vi "From Notification Key.vi"(2 "Key":string) -> (5 "Alias":string, 8 "Symbol Name":string)   [LabVIEW 2018, in "TwinCAT ADS.lvclass"]
uses:
  TwinCAT ADS.lvclass
  Controls/ADS Notification Map Key.ctl
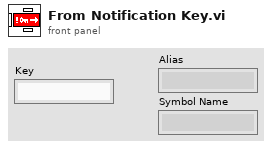
[diagram p1: front panel]
types:
  T1 = typedef "TwinCAT ADS.lvclass/ADS Notification Map Key.ctl" = cluster{"Alias":string, "Symbol Name":string}
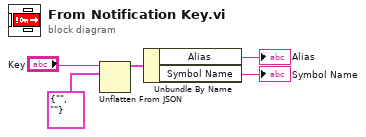
[diagram p0: block diagram]
diagram:
  n1 = Unflatten From JSON(JSON string="Key", type and defaults=T1 {"Alias"="", "Symbol Name"=""} ("Notification User Data")) -> (value=w3:T1)  [unwired: 5 in, 1 out]
  n2 = Unbundle By Name(w3) -> ("Alias"=→"Alias":string, "Symbol Name"=→"Symbol Name":string)
